vi "Pre Launch Init.vi"(11 "Simulated Dual Fan":refnum<class "Simulated Dual Fan.lvclass">) -> (0 "error out":errorcluster, 3 "Simulated Dual Fan":refnum<class "Simulated Dual Fan.lvclass">)   [LabVIEW 2025, in "Simulated Dual Fan.lvclass"]
uses:
  Simulated Dual Fan.lvclass
  Cooler Plug-Ins/Simulated Evaporative Cooler.lvclass/Simulation Data_Global.vi
  Dual Fan/Dual Fan/Dual Fan.lvclass
  Cooler Plug-Ins/Simulated Evaporative Cooler.lvclass/Simulated Evaporative Cooler.lvclass
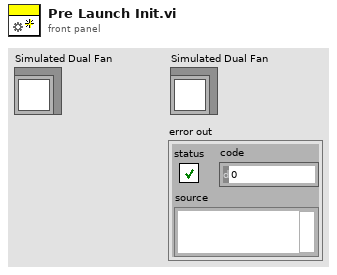
[diagram p1: front panel]
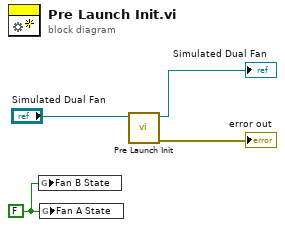
[diagram p0: block diagram]
diagram:
  w2 = FALSE
  n1 = global write "Simulation Data_Global.vi" "Fan B State"(w2) -> ()
  n2 = global write "Simulation Data_Global.vi" "Fan A State"(w2) -> ()
  n3 = call-parent "Pre Launch Init.vi"("Timed Loop Controller in"="Simulated Dual Fan") -> ("error out"=→"error out":errorcluster, "Timed Loop Controller out"=→"Simulated Dual Fan":refnum<class "Simulated Dual Fan.lvclass">)  [unwired: 9 in]
